vi "ProfiledPIDController_SetPID.vi"(8 "Kd":dbl, 9 "Ki":dbl, 10 "Kp":dbl, 11 "in PROFILED_PID_CONTROLLER":T1={"Controller"={"Kp"=0.0, "Ki"=0.0, "Kd"=0.0, "Period"=0.0, "Max_Integral"=1.0, "Min_Integral"=-1.0, "Max_Input"=0.0, "Min_Input"=0.0, "Continuous"=FALSE, "PositionError"=0.0, "VelocityError"=0.0, "PrevError"=0.0, "TotalError"=0.0, "PositionTolerance"=0.05, "VelocityTolerance"=9.99e+35, "SetPoint"=0.0, "Kf"=0.0, "Prev_Deriv"=0.0, "Prev_Deriv 2"=0.0, "DerivativeFilter"=FALSE, "Min_Output"=-9.99e+35, "Max_Output"=9.9e+35, "Prev_F_P"=0.0, "Prev_F_P_2"=0.0, "AntiWindupActive"=FALSE}, "Goal"={"Position"=0.0, "Velocity"=0.0}, "Setpoint"={"Position"=0.0, "Velocity"=0.0}, "Constraint"={"MaxVelocity"=0.0, "MaxAcceleration"=0.0}} {"Constraint"."MaxAcceleration" format="%16_6e"; "Constraint"."MaxVelocity" format="%16_6e"; "Setpoint"."Velocity" format="%16_6e"; "Setpoint"."Position" format="%16_6e"; "Goal"."Velocity" format="%16_6e"; "Goal"."Position" format="%16_6e"; "Controller"."Prev_F_P_2" format="%16_6e"; "Controller"."Prev_F_P" format="%16_6e"; "Controller"."Max_Output" format="%16_6e"; "Controller"."Min_Output" format="%16_6e"; "Controller"."Prev_Deriv 2" format="%16_6e"; "Controller"."Prev_Deriv" format="%16_6e"; "Controller"."Kf" format="%16_6e"; "Controller"."SetPoint" format="%16_6e"; "Controller"."VelocityTolerance" format="%16_6e"; "Controller"."PositionTolerance" format="%16_6e"; "Controller"."TotalError" format="%16_6e"; "Controller"."PrevError" format="%16_6e"; "Controller"."VelocityError" format="%16_6e"; "Controller"."PositionError" format="%16_6e"; "Controller"."Min_Input" format="%16_6e"; "Controller"."Max_Input" format="%16_6e"; "Controller"."Min_Integral" format="%16_6e"; "Controller"."Max_Integral" format="%16_6e"; "Controller"."Period" format="%16_6e"; "Controller"."Kd" format="%16_6e"; "Controller"."Ki" format="%16_6e"; "Controller"."Kp" format="%16_6e"}) -> (3 "out PROFILED_PID_CONTROLLER":T1={"Controller"={"Kp"=0.0, "Ki"=0.0, "Kd"=0.0, "Period"=0.0, "Max_Integral"=1.0, "Min_Integral"=-1.0, "Max_Input"=0.0, "Min_Input"=0.0, "Continuous"=FALSE, "PositionError"=0.0, "VelocityError"=0.0, "PrevError"=0.0, "TotalError"=0.0, "PositionTolerance"=0.05, "VelocityTolerance"=9.99e+35, "SetPoint"=0.0, "Kf"=0.0, "Prev_Deriv"=0.0, "Prev_Deriv 2"=0.0, "DerivativeFilter"=FALSE, "Min_Output"=-9.99e+35, "Max_Output"=9.9e+35, "Prev_F_P"=0.0, "Prev_F_P_2"=0.0, "AntiWindupActive"=FALSE}, "Goal"={"Position"=0.0, "Velocity"=0.0}, "Setpoint"={"Position"=0.0, "Velocity"=0.0}, "Constraint"={"MaxVelocity"=0.0, "MaxAcceleration"=0.0}} {"Constraint"."MaxAcceleration" format="%16_6e"; "Constraint"."MaxVelocity" format="%16_6e"; "Setpoint"."Velocity" format="%16_6e"; "Setpoint"."Position" format="%16_6e"; "Goal"."Velocity" format="%16_6e"; "Goal"."Position" format="%16_6e"; "Controller"."Prev_F_P_2" format="%16_6e"; "Controller"."Prev_F_P" format="%16_6e"; "Controller"."Max_Output" format="%16_6e"; "Controller"."Min_Output" format="%16_6e"; "Controller"."Prev_Deriv 2" format="%16_6e"; "Controller"."Prev_Deriv" format="%16_6e"; "Controller"."Kf" format="%16_6e"; "Controller"."SetPoint" format="%16_6e"; "Controller"."VelocityTolerance" format="%16_6e"; "Controller"."PositionTolerance" format="%16_6e"; "Controller"."TotalError" format="%16_6e"; "Controller"."PrevError" format="%16_6e"; "Controller"."VelocityError" format="%16_6e"; "Controller"."PositionError" format="%16_6e"; "Controller"."Min_Input" format="%16_6e"; "Controller"."Max_Input" format="%16_6e"; "Controller"."Min_Integral" format="%16_6e"; "Controller"."Max_Integral" format="%16_6e"; "Controller"."Period" format="%16_6e"; "Controller"."Kd" format="%16_6e"; "Controller"."Ki" format="%16_6e"; "Controller"."Kp" format="%16_6e"})   [LabVIEW 2019, in "Trajectory_Library.lvlib"]
doc: "Sets the PID Controller gain parameters.\n\nSets the proportional, integral, and differential coefficients.\n\nInputs:\n - Profiled_PID_Controller -- Profiled_PID_Controller data cluster\n - Kp -- Proportional coefficient\n - Ki -- Integral coefficient\n - Kd -- Differential coefficient\n\nOutputs:\n - Profiled_PID_Controller -- Updated Profiled_PID_Controller data cluster"
uses:
  Trajectory_Library.lvlib
  PROFILED_PID_CONTROLLER.ctl
  PID_CONTROLLER.ctl
  TRAPEZOID_PROFILE_STATE.ctl
  TRAPEZOID_PROFILE_CONSTRAINT.ctl
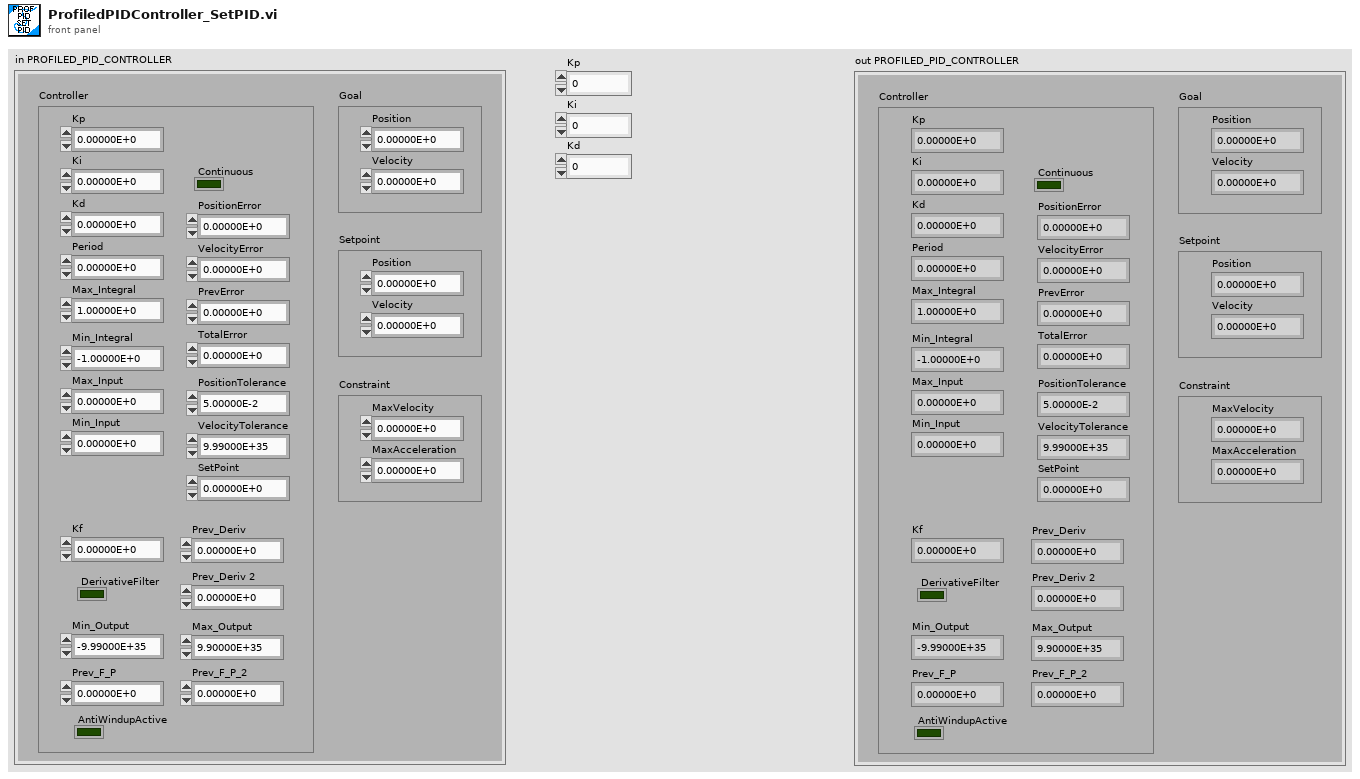
[diagram p1: front panel]
types:
  T1 = typedef "Trajectory_Library.lvlib/PROFILED_PID_CONTROLLER.ctl" = cluster{"Controller":T2, "Goal":T3, "Setpoint":T3, "Constraint":T4}
  T2 = typedef "Trajectory_Library.lvlib/PID_CONTROLLER.ctl" = cluster{"Kp":dbl, "Ki":dbl, "Kd":dbl, "Period":dbl, "Max_Integral":dbl, "Min_Integral":dbl, "Max_Input":dbl, "Min_Input":dbl, "Continuous":bool, "PositionError":dbl, "VelocityError":dbl, "PrevError":dbl, "TotalError":dbl, "PositionTolerance":dbl, "VelocityTolerance":dbl, "SetPoint":dbl, "Kf":dbl, "Prev_Deriv":dbl, "Prev_Deriv 2":dbl, "DerivativeFilter":bool, "Min_Output":dbl, "Max_Output":dbl, "Prev_F_P":dbl, "Prev_F_P_2":dbl, "AntiWindupActive":bool}
  T3 = typedef "Trajectory_Library.lvlib/TRAPEZOID_PROFILE_STATE.ctl" = cluster{"Position":dbl, "Velocity":dbl}
  T4 = typedef "Trajectory_Library.lvlib/TRAPEZOID_PROFILE_CONSTRAINT.ctl" = cluster{"MaxVelocity":dbl, "MaxAcceleration":dbl}
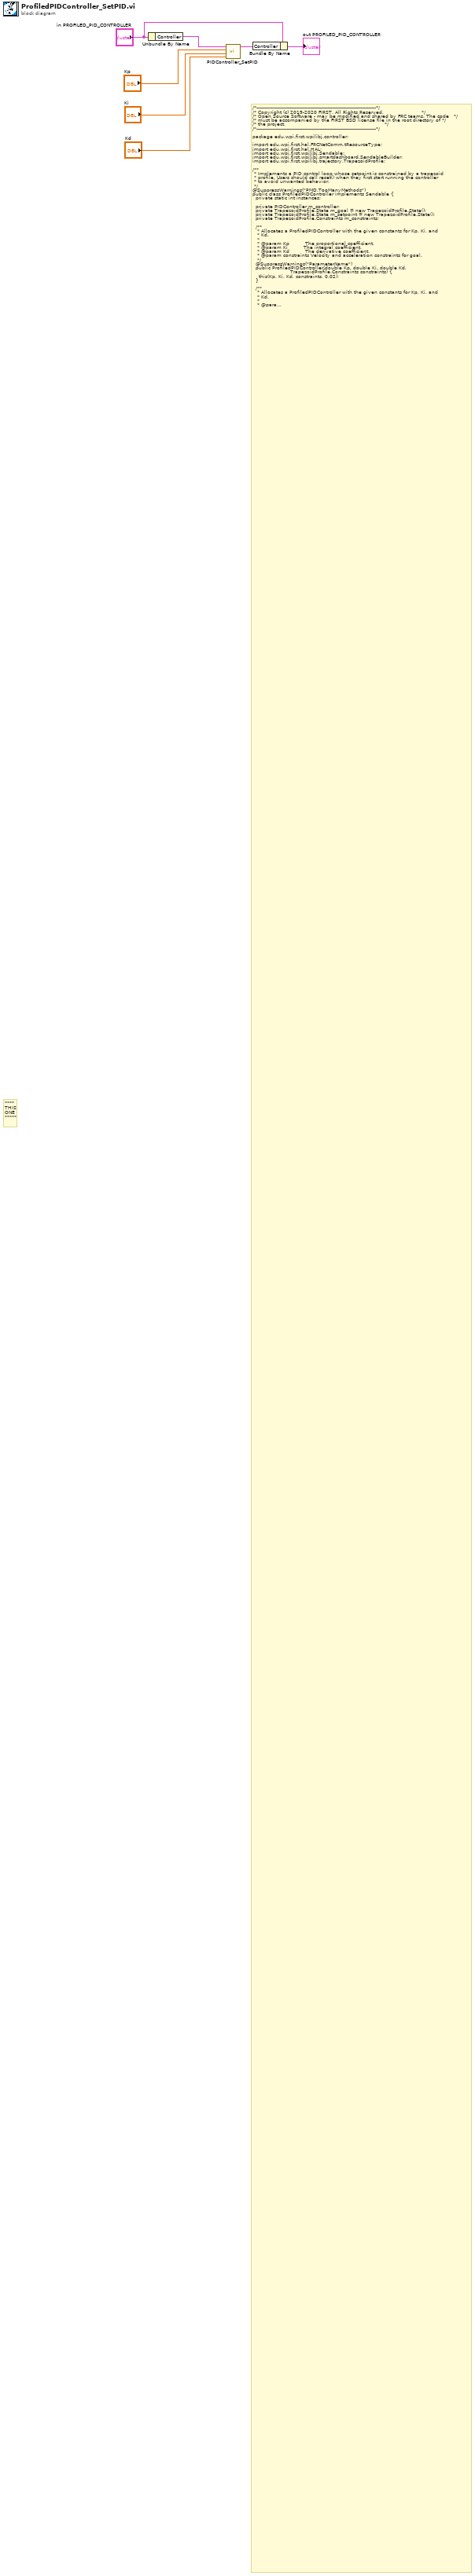
[diagram p0: block diagram]
diagram:
  # "/*----------------------------------------------------------------------------*/\n/* Copyright (c) 2019-2020 FIRST. All Rights Reserved.                        */\n/* Open Source Software - may be modified and shared by FRC teams. The code   */\n/* must be accompanied by the FIRST BSD license file in the root directory of */\n/* the project.                                                               */\n/*----------------------------------------------------------------------------*/\n\npackage edu.wpi.first.wpilibj.controller;\n\nimport edu.wpi.first.hal.FRCNetComm.tResourceType;\nimport edu.wpi.first.hal.HAL;\nimport edu.wpi.first.wpilibj.Sendable;\nimport edu.wpi.first.wpilibj.smartdashboard.SendableBuilder;\nimport edu.wpi.first.wpilibj.trajectory.TrapezoidProfile;\n\n/**\n * Implements a PID control loop whose setpoint is constrained by a trapezoid\n * profile. Users should call reset() when they first start running the controller\n * to avoid unwanted behavior.\n */\n@SuppressWarnings(\"PMD.TooManyMethods\")\npublic class ProfiledPIDController implements Sendable {\n  private static int instances;\n\n  private PIDController m_controller;\n  private TrapezoidProfile.State m_goal = new TrapezoidProfile.State();\n  private TrapezoidProfile.State m_setpoint = new TrapezoidProfile.State();\n  private TrapezoidProfile.Constraints m_constraints;\n\n  /**\n   * Allocates a ProfiledPIDController with the given constants for Kp, Ki, and\n   * Kd.\n   *\n   * @param Kp          The proportional coefficient.\n   * @param Ki          The integral coefficient.\n   * @param Kd          The derivative coefficient.\n   * @param constraints Velocity and acceleration constraints for goal.\n   */\n  @SuppressWarnings(\"ParameterName\")\n  public ProfiledPIDController(double Kp, double Ki, double Kd,\n                        TrapezoidProfile.Constraints constraints) {\n    this(Kp, Ki, Kd, constraints, 0.02);\n  }\n\n  /**\n   * Allocates a ProfiledPIDController with the given constants for Kp, Ki, and\n   * Kd.\n   *\n   * @param Kp          The proportional coefficient.\n   * @param Ki          The integral coefficient.\n   * @param Kd          The derivative coefficient.\n   * @param constraints Velocity and acceleration constraints for goal.\n   * @param period      The period between controller updates in seconds. The\n   *                    default is 0.02 seconds.\n   */\n  @SuppressWarnings(\"ParameterName\")\n  public ProfiledPIDController(double Kp, double Ki, double Kd,\n                        TrapezoidProfile.Constraints constraints,\n                        double period) {\n    m_controller = new PIDController(Kp, Ki, Kd, period);\n    m_constraints = constraints;\n    instances++;\n    HAL.report(tResourceType.kResourceType_ProfiledPIDController, instances);\n  }\n\n  /**\n   * Sets the PID Controller gain parameters.\n   *\n   * <p>Sets the proportional, integral, and differential coefficients.\n   *\n   * @param Kp Proportional coefficient\n   * @param Ki Integral coefficient\n   * @param Kd Differential coefficient\n   */\n  @SuppressWarnings(\"ParameterName\")\n  public void setPID(double Kp, double Ki, double Kd) {\n    m_controller.setPID(Kp, Ki, Kd);\n  }\n\n  /**\n   * Sets the proportional coefficient of the PID controller gain.\n   *\n   * @param Kp proportional coefficient\n   */\n  @SuppressWarnings(\"ParameterName\")\n  public void setP(double Kp) {\n    m_controller.setP(Kp);\n  }\n\n  /**\n   * Sets the integral coefficient of the PID controller gain.\n   *\n   * @param Ki integral coefficient\n   */\n  @SuppressWarnings(\"ParameterName\")\n  public void setI(double Ki) {\n    m_controller.setI(Ki);\n  }\n\n  /**\n   * Sets the differential coefficient of the PID controller gain.\n   *\n   * @param Kd differential coefficient\n   */\n  @SuppressWarnings(\"ParameterName\")\n  public void setD(double Kd) {\n    m_controller.setD(Kd);\n  }\n\n  /**\n   * Gets the proportional coefficient.\n   *\n   * @return proportional coefficient\n   */\n  public double getP() {\n    return m_controller.getP();\n  }\n\n  /**\n   * Gets the integral coefficient.\n   *\n   * @return integral coefficient\n   */\n  public double getI() {\n    return m_controller.getI();\n  }\n\n  /**\n   * Gets the differential coefficient.\n   *\n   * @return differential coefficient\n   */\n  public double getD() {\n    return m_controller.getD();\n  }\n\n  /**\n   * Gets the period of this controller.\n   *\n   * @return The period of the controller.\n   */\n  public double getPeriod() {\n    return m_controller.getPeriod();\n  }\n\n  /**\n   * Sets the goal for the ProfiledPIDController.\n   *\n   * @param goal The desired goal state.\n   */\n  public void setGoal(TrapezoidProfile.State goal) {\n    m_goal = goal;\n  }\n\n  /**\n   * Sets the goal for the ProfiledPIDController.\n   *\n   * @param goal The desired goal position.\n   */\n  public void setGoal(double goal) {\n    m_goal = new TrapezoidProfile.State(goal, 0);\n  }\n\n  /**\n   * Gets the goal for the ProfiledPIDController.\n   */\n  public TrapezoidProfile.State getGoal() {\n    return m_goal;\n  }\n\n  /**\n   * Returns true if the error is within the tolerance of the error.\n   *\n   * <p>This will return false until at least one input value has been computed.\n   */\n  public boolean atGoal() {\n    return atSetpoint() && m_goal.equals(m_setpoint);\n  }\n\n  /**\n   * Set velocity and acceleration constraints for goal.\n   *\n   * @param constraints Velocity and acceleration constraints for goal.\n   */\n  public void setConstraints(TrapezoidProfile.Constraints constraints) {\n    m_constraints = constraints;\n  }\n\n  /**\n   * Returns the current setpoint of the ProfiledPIDController.\n   *\n   * @return The current setpoint.\n   */\n  public TrapezoidProfile.State getSetpoint() {\n    return m_setpoint;\n  }\n\n  /**\n   * Returns true if the error is within the tolerance of the error.\n   *\n   * <p>This will return false until at least one input value has been computed.\n   */\n  public boolean atSetpoint() {\n    return m_controller.atSetpoint();\n  }\n\n  /**\n   * Enables continuous input.\n   *\n   * <p>Rather then using the max and min input range as constraints, it considers\n   * them to be the same point and automatically calculates the shortest route\n   * to the setpoint.\n   *\n   * @param minimumInput The minimum value expected from the input.\n   * @param maximumInput The maximum value expected from the input.\n   */\n  public void enableContinuousInput(double minimumInput, double maximumInput) {\n    m_controller.enableContinuousInput(minimumInput, maximumInput);\n  }\n\n  /**\n   * Disables continuous input.\n   */\n  public void disableContinuousInput() {\n    m_controller.disableContinuousInput();\n  }\n\n  /**\n   * Sets the minimum and maximum values for the integrator.\n   *\n   * <p>When the cap is reached, the integrator value is added to the controller\n   * output rather than the integrator value times the integral gain.\n   *\n   * @param minimumIntegral The minimum value of the integrator.\n   * @param maximumIntegral The maximum value of the integrator.\n   */\n  public void setIntegratorRange(double minimumIntegral, double maximumIntegral) {\n    m_controller.setIntegratorRange(minimumIntegral, maximumIntegral);\n  }\n\n  /**\n   * Sets the error which is considered tolerable for use with atSetpoint().\n   *\n   * @param positionTolerance Position error which is tolerable.\n   */\n  public void setTolerance(double positionTolerance) {\n    setTolerance(positionTolerance, Double.POSITIVE_INFINITY);\n  }\n\n  /**\n   * Sets the error which is considered tolerable for use with atSetpoint().\n   *\n   * @param positionTolerance Position error which is tolerable.\n   * @param velocityTolerance Velocity error which is tolerable.\n   */\n  public void setTolerance(double positionTolerance, double velocityTolerance) {\n    m_controller.setTolerance(positionTolerance, velocityTolerance);\n  }\n\n  /**\n   * Returns the difference between the setpoint and the measurement.\n   *\n   * @return The error.\n   */\n  public double getPositionError() {\n    return m_controller.getPositionError();\n  }\n\n  /**\n   * Returns the change in error per second.\n   */\n  public double getVelocityError() {\n    return m_controller.getVelocityError();\n  }\n\n  /**\n   * Returns the next output of the PID controller.\n   *\n   * @param measurement The current measurement of the process variable.\n   */\n  public double calculate(double measurement) {\n    var profile = new TrapezoidProfile(m_constraints, m_goal, m_setpoint);\n    m_setpoint = profile.calculate(getPeriod());\n    return m_controller.calculate(measurement, m_setpoint.position);\n  }\n\n  /**\n   * Returns the next output of the PID controller.\n   *\n   * @param measurement The current measurement of the process variable.\n   * @param goal The new goal of the controller.\n   */\n  public double calculate(double measurement, TrapezoidProfile.State goal) {\n    setGoal(goal);\n    return calculate(measurement);\n  }\n\n  /**\n   * Returns the next output of the PIDController.\n   *\n   * @param measurement The current measurement of the process variable.\n   * @param goal The new goal of the controller.\n   */\n  public double calculate(double measurement, double goal) {\n    setGoal(goal);\n    return calculate(measurement);\n  }\n\n  /**\n   * Returns the next output of the PID controller.\n   *\n   * @param measurement The current measurement of the process variable.\n   * @param goal        The new goal of the controller.\n   * @param constraints Velocity and acceleration constraints for goal.\n   */\n  public double calculate(double measurement, TrapezoidProfile.State goal,\n                   TrapezoidProfile.Constraints constraints) {\n    setConstraints(constraints);\n    return calculate(measurement, goal);\n  }\n\n  /**\n   * Reset the previous error and the integral term.\n   *\n   * @param measurement The current measured State of the system.\n   */\n  public void reset(TrapezoidProfile.State measurement) {\n    m_controller.reset();\n    m_setpoint = measurement;\n  }\n\n  /**\n   * Reset the previous error and the integral term.\n   *\n   * @param measuredPosition The current measured position of the system.\n   * @param measuredVelocity The current measured velocity of the system.\n   */\n  public void reset(double measuredPosition, double measuredVelocity) {\n    reset(new TrapezoidProfile.State(measuredPosition, measuredVelocity));\n  }\n\n  /**\n   * Reset the previous error and the integral term.\n   *\n   * @param measuredPosition The current measured position of the system. The velocity is\n   *     assumed to be zero.\n   */\n  public void reset(double measuredPosition) {\n    reset(measuredPosition, 0.0);\n  }\n\n  @Override\n  public void initSendable(SendableBuilder builder) {\n    builder.setSmartDashboardType(\"ProfiledPIDController\");\n    builder.addDoubleProperty(\"p\", this::getP, this::setP);\n    builder.addDoubleProperty(\"i\", this::getI, this::setI);\n    builder.addDoubleProperty(\"d\", this::getD, this::setD);\n    builder.addDoubleProperty(\"goal\", () -> getGoal().position, this::setGoal);\n  }\n}"
  # "****\nTHIS\nONE\n*****"
  n1 = Unbundle By Name("in PROFILED_PID_CONTROLLER") -> ("Controller"=w4:T2)
  n2 = call "PIDController_SetPID.vi"("Kd"="Kd", "Ki"="Ki", "Kp"="Kp", "in PID_CONTROLLER"=w4) -> ("out PID_CONTROLLER"=w5:T2)  [unwired: 7 in]
  n3 = Bundle By Name(cluster="in PROFILED_PID_CONTROLLER", "Controller"=w5) -> (→"out PROFILED_PID_CONTROLLER":T1)
